vi "BeepWrapper2.vi"   [LabVIEW 2026]
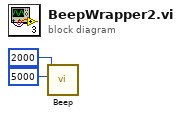
[diagram p0: block diagram]
diagram:
  n1 = call <vilib>:"Beep.vi"("duration (msec)"=u32 5000, "frequency (Hz)"=u32 2000) -> ()  [unwired: 10 in]
